vi "Analog Output.vi"() -> ()   [LabVIEW 2016]
doc: "This VI will continually write single point values to 4 channels."
uses:
  <vilib>/eio/EIONode/EIONode.xnode
  <vilib>/rvi/eio/common/nirviEmuTemplateMethod_errors.vi
panel:
  in  "Loop Rate (uS)":u32=10
  in  "AO Data":T1
  # "Overview: Demonstrates the use of the analog output FPGA I/O on R Series devices.\nRequirements: LabVIEW FPGA Module, NI-RIO\nInstructions: \nRun the VI."
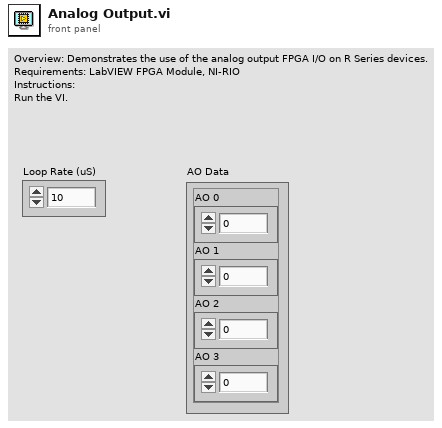
[diagram p1: front panel]
types:
  T1 = cluster{"AO 0":i16, "AO 1":i16, "AO 2":i16, "AO 3":i16}
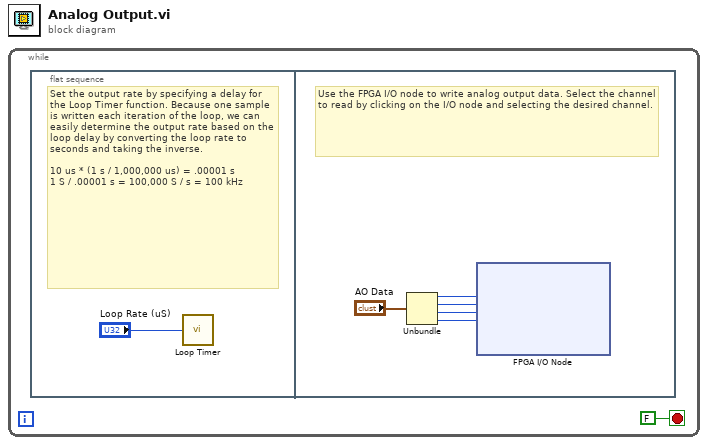
[diagram p0: block diagram]
diagram:
  n1 = while {
    stop <- FALSE ("Stop") stop-if-true
    # "Main Processing Loop"
    n2 = flat-sequence {
      frame #0 {
        # "Set the output rate by specifying a delay for the Loop Timer function. Because one sample is written each iteration of the loop, we can easily determine the output rate based on the loop delay by converting the loop rate to seconds and taking the inverse. \n\n10 us * (1 s / 1,000,000 us) = .00001 s\n1 S / .00001 s = 100,000 S / s = 100 kHz"
        n3 = call "Loop Timer"("Count(uSec)"="Loop Rate (uS)") -> ()  [unwired: 1 out]
      }
      frame #1 {
        # "Use the FPGA I/O node to write analog output data. Select the channel to read by clicking on the I/O node and selecting the desired channel."
        n4 = Unbundle("AO Data") -> ("AO 0"=w4:i16, "AO 1"=w5:i16, "AO 2"=w6:i16, "AO 3"=w7:i16)
        n5 = xnode "FPGA I/O Node"("Connector0/AO0"=w4, "Connector0/AO1"=w5, "Connector0/AO2"=w6, "Connector0/AO3"=w7) -> ()  [unwired: 5 in, 5 out]
      }
    }
  }
